vi "Dopocet_presne_nuly.vi"(8 "dt":dbl, 11 "Vstupní pole":dbl[](array[numeric])) -> (2 "XY Graph":cluster{dbl[], "Vstupní pole":dbl[]}(graph))   [LabVIEW 2019]
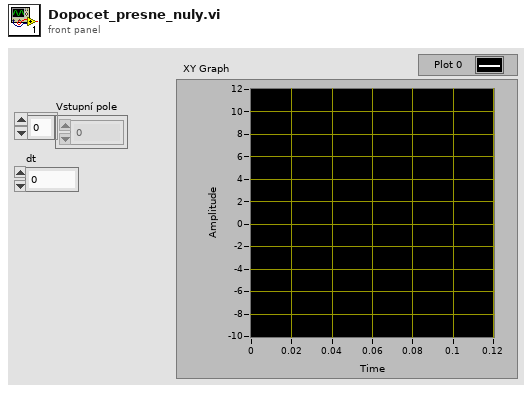
[diagram p1: front panel]
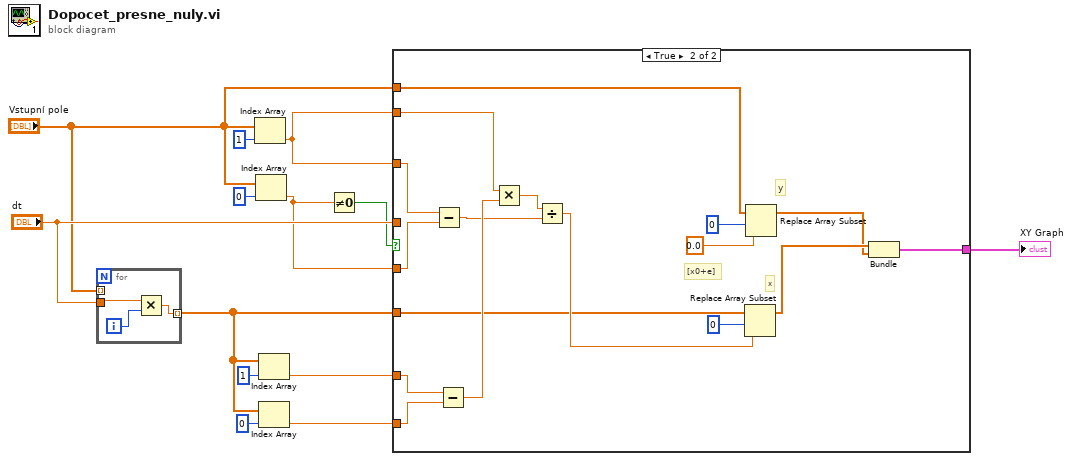
[diagram p0: block diagram]
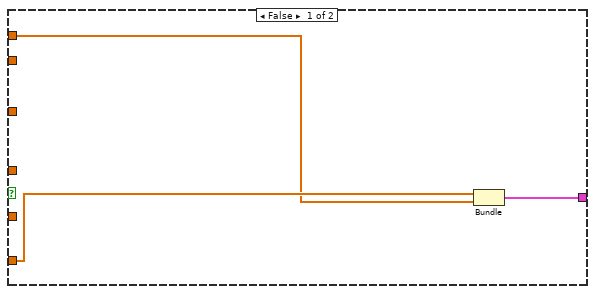
[diagram p2: hidden frame]
diagram:
  n1 = for {
    tunnel: "dt" -> [w15]
    tunnel: "Vstupní pole" -> [_] mode=indexing
    tunnel: [w14] -> w6 mode=indexing
    i -> [w16]
    n2 = Multiply(x=w15, y=w16) -> (x*y=w14:dbl)
  }
  n3 = Index Array(array="Vstupní pole", index=1) -> (element=w3:dbl)
  n4 = Index Array(array="Vstupní pole", index=0) -> (element=w10:dbl)
  n5 = Index Array(array=w6, index=1) -> (element=w5:dbl)
  n6 = Index Array(array=w6, index=0) -> (element=w4:dbl)
  n7 = Not Equal To 0?(x=w10) -> (x != 0?=w9:bool)
  n8 = case shown="True" w9 {
    tunnel: w3 -> [_ w30]
    tunnel: w10 -> [_ w29]
    tunnel: "dt" -> [_ _]
    tunnel: w3 -> [_ w20]
    tunnel: w6 -> [w19 w21]
    tunnel: w5 -> [_ w31]
    tunnel: w4 -> [_ w28]
    tunnel: [w18 w23] -> w2
    tunnel: "Vstupní pole" -> [w17 w22]
    frame False {
      n9 = Bundle(w19, "Vstupní pole"=w17) -> (w18:cluster{dbl[], "Vstupní pole":dbl[]})  [unwired: 1 in]
    }
    frame True {
      # "x"
      # "y"
      # "[x0+e]"
      n10 = Subtract(x=w30, y=w29) -> (x-y=w25:dbl)
      n11 = Subtract(x=w31, y=w28) -> (x-y=w27:dbl)
      n12 = Multiply(x=w20, y=w27) -> (x*y=w26:dbl)
      n13 = Divide(x=w26, y=w25) -> (x/y=w24:dbl)
      n14 = Replace Array Subset(array=w21, new element=w24, index=0) -> (w33:dbl[])
      n15 = Replace Array Subset(array=w22, new element=0.0, index=0) -> (w32:dbl[])
      n16 = Bundle(w33, "Vstupní pole"=w32) -> (w23:cluster{dbl[], "Vstupní pole":dbl[]})  [unwired: 1 in]
    }
  }
  "XY Graph" <- w2
